vi "Enqueue Message.vi"   [LabVIEW 2018, in "Message Queue.lvlib"]
doc: "일반 메시지의 경우, 메시지를 큐에 추가합니다. 우선순위 메시지의 경우, 메시지를 큐의 앞쪽에 추가합니다."
uses:
  Message Queue.lvlib
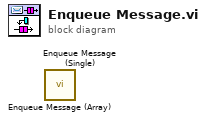
[diagram p0: block diagram]
diagram:
  n1 = call "Enqueue Message (Array).vi"() -> ()  [unwired: 10 in, 2 out]
  n2 = call "Enqueue Message (Single).vi"() -> ()  [unwired: 10 in, 2 out]
